vi "Laboratory_practice12.vi"() -> ()   [LabVIEW 2021]
uses:
  <vilib>/Waveform/WDTFileIO.llb/Export Waveforms To Spreadsheet File (1D).vi
panel:
  in  "rate":dbl=5000.0
  in  "number of samples":i32=100
  out "data":dynamicdata(graph)
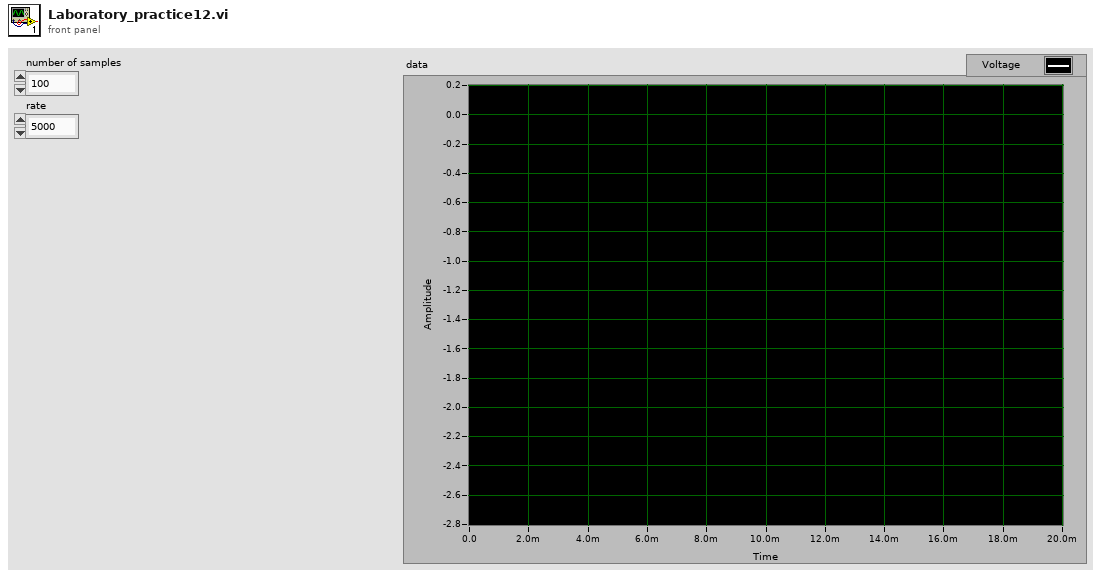
[diagram p1: front panel]
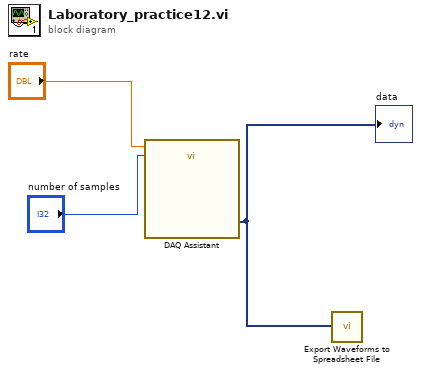
[diagram p0: block diagram]
diagram:
  n1 = call "DAQ Assistant"("rate"="rate", "number of samples"="number of samples") -> ("data"=w1:dynamicdata)  [unwired: 15 in, 2 out]
  "data" <- w1
  n2 = call-poly <vilib>:"Export Waveforms to Spreadsheet File.vi"("waveforms"=w1) -> ()  [unwired: 9 in, 2 out]
